vi "Error Handler - Acquisition Message Loop.vi"(8 "error in (no error)":errorcluster, 9 "Motor":refnum<queue>, 10 "Ignore Errors (Runtime)":i32[](array[numeric]), 11 "Message Queue":refnum<queue>) -> (0 "dup error in":errorcluster, 3 "dup Message Queue":refnum<queue>)   [LabVIEW 2020, in "MOTOR.lvlib"]
doc: "Process an error that occurred in the Acquisition Message Loop, either by ignoring it, or generating an \"Error\" message."
uses:
  MOTOR.lvlib
  support/Message Queue/Message Cluster.ctl
  support/Message Queue/Enqueue Message (Single).vi
  support/Message Queue/Message Queue.lvlib
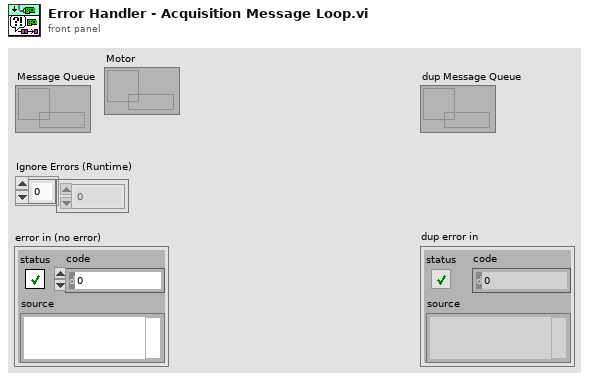
[diagram p1: front panel]
types:
  T1 = typedef "Message Queue.lvlib/Message Cluster.ctl" = cluster{"Message":string, "Message Data":variant}
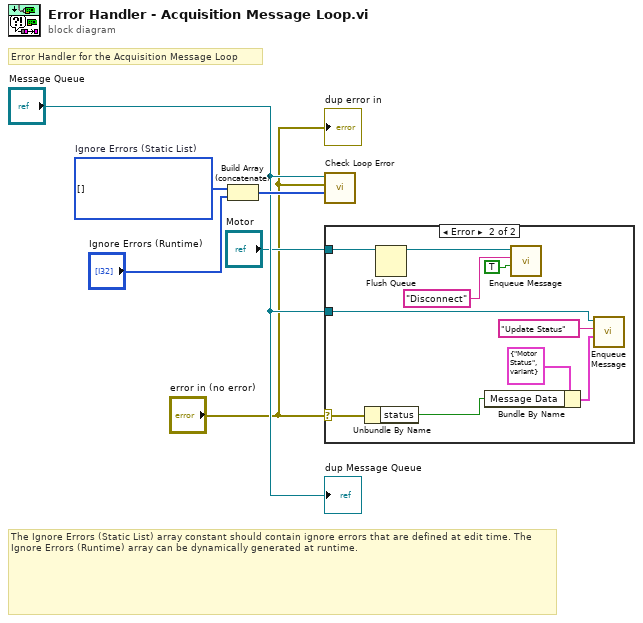
[diagram p0: block diagram]
diagram:
  w6 = i32[] []  # Ignore Errors (Static List)
  # "The Ignore Errors (Static List) array constant should contain ignore errors that are defined at edit time. The Ignore Errors (Runtime) array can be dynamically generated at runtime."
  # "Error Handler for the Acquisition Message Loop"
  n1 = Build Array (concatenate)(w6, "Ignore Errors (Runtime)") -> (w4:i32[])
  n2 = call "Check Loop Error.vi"("Ignore Errors"=w4, "error to process"="error in (no error)", "Message Queue"="Message Queue") -> ()  [unwired: 7 in, 2 out]
  n3 = case shown="Error" "error in (no error)" {
    selector: "error in (no error)" -> [_ w11]
    tunnel: "Message Queue" -> [_ w12]
    tunnel: "Motor" -> [_ w8]
    frame No Error {
    }
    frame Error {
      n4 = Unbundle By Name(w11) -> ("status"=w15:bool)
      n5 = Flush Queue(queue=w8) -> (queue out=w7:refnum<queue>)  [unwired: 1 in, 2 out]
      n6 = Bundle By Name(cluster=T1 {"Message"="Motor Status", "Message Data"=variant} ("Message Cluster"), "Message Data"=w15) -> (w14:T1)
      n7 = call-poly "Enqueue Message.vi"("Message Data"=TRUE, "Message"="Disconnect", "Message Queue"=w7) -> ()  [unwired: 7 in, 2 out]
      n8 = call-poly "Enqueue Message.vi"("Message Data"=w14, "Message"="Update Status", "Message Queue"=w12) -> ()  [unwired: 7 in, 2 out]
    }
  }
  "dup Message Queue" <- "Message Queue"
  "dup error in" <- "error in (no error)"
